vi "LinearMap.vi"(0 "Criterion in":refnum<class "Criterion.lvclass">, 1 "MaxEvalutation":dbl, 5 "MaxVal":dbl, 7 "Val":dbl, 9 "MinVal":dbl, 11 "error in (no error)":errorcluster, 12 "MinEvaluation":dbl) -> (4 "Criterion out":refnum<class "Criterion.lvclass">, 8 "Evaluation":dbl, 15 "error out":errorcluster)   [LabVIEW 2023, in "Criterion.lvclass"]
uses:
  Criterion.lvclass
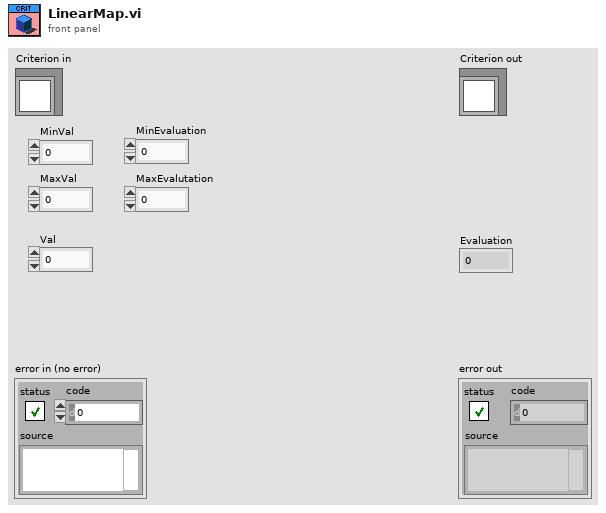
[diagram p1: front panel]
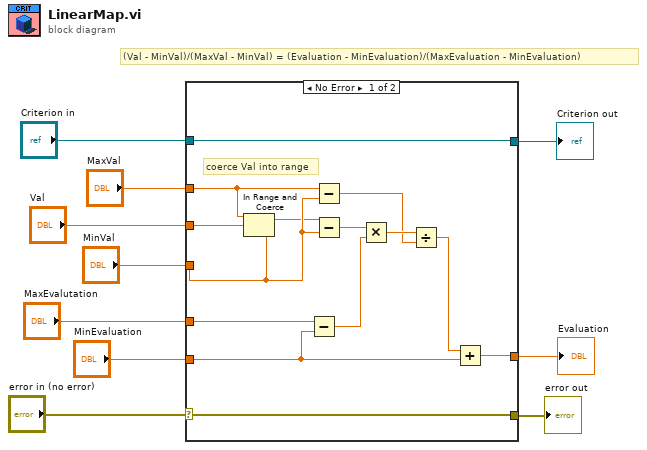
[diagram p0: block diagram]
diagram:
  # "(Val - MinVal)/(MaxVal - MinVal) = (Evaluation - MinEvaluation)/(MaxEvaluation - MinEvaluation)"
  n1 = case shown="No Error" "error in (no error)" {
    selector: "error in (no error)" -> [w23 w26]
    tunnel: [w23 w26] -> w9
    tunnel: [w24 w25] -> w7
    tunnel: "Criterion in" -> [w24 w25]
    tunnel: "MaxEvalutation" -> [w21 _]
    tunnel: "MinEvaluation" -> [w20 _]
    tunnel: "MinVal" -> [w12 _]
    tunnel: "Val" -> [w14 _]
    tunnel: "MaxVal" -> [w13 _]
    tunnel: [w22 _] -> w1
    frame No Error {
      # "coerce Val into range"
      n2 = In Range and Coerce(upper limit=w13, x=w14, lower limit=w12) -> (coerced(x)=w11:dbl)  [unwired: 1 out]
      n3 = Subtract(x=w21, y=w20) -> (x-y=w19:dbl)
      n4 = Subtract(x=w13, y=w12) -> (x-y=w16:dbl)
      n5 = Subtract(x=w11, y=w12) -> (x-y=w18:dbl)
      n6 = Multiply(x=w18, y=w19) -> (x*y=w17:dbl)
      n7 = Divide(x=w17, y=w16) -> (x/y=w15:dbl)
      n8 = Add(x=w15, y=w20) -> (x+y=w22:dbl)
    }
    frame Error {
    }
  }
  "error out" <- w9
  "Criterion out" <- w7
  "Evaluation" <- w1
